vi "Frame_Packet.vi"(10 "String in":string, 11 "Numeric in":u32) -> (2 "Numeric out":i32, 3 "String out":string)   [LabVIEW 2017]
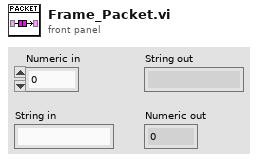
[diagram p1: front panel]
types:
  T1 = enum16{"big-endian, network order", "native, host order", "little-endian"}
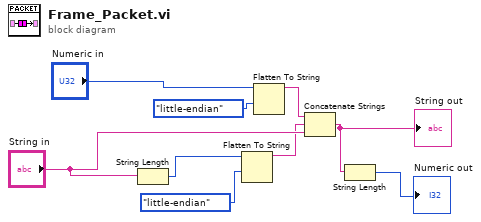
[diagram p0: block diagram]
diagram:
  n1 = String Length(string="String in") -> (length=w1:i32)
  n2 = Flatten To String(anything=w1, byte order (0:big-endian, network order)=T1."little-endian") -> (data string=w3:string)  [unwired: 2 in, 2 out]
  n3 = Flatten To String(anything="Numeric in", byte order (0:big-endian, network order)=T1."little-endian") -> (data string=w8:string)  [unwired: 2 in, 2 out]
  n4 = Concatenate Strings(w8, w3, "String in") -> (w6:string)
  "String out" <- w6
  n5 = String Length(string=w6) -> (length=→"Numeric out":i32)
